vi "Move To Abs.vi"(8 "error in (no error)":errorcluster, 9 "Step In range":bool, 10 "Possition selector":T1(radio), 11 "Lifter_motor in":refnum<class "Lifter_motor.lvclass">) -> (0 "error out":errorcluster, 3 "Lifter_motor out":refnum<class "Lifter_motor.lvclass">)   [LabVIEW 2019, in "Lifter_motor.lvclass"]
uses:
  Lifter_motor.lvclass
  Lifter_motor.lvclass/Lifter_motor.ctl
  TCP Class/LifterTCP.lvclass
panel:
  out "Driver ACK?":bool
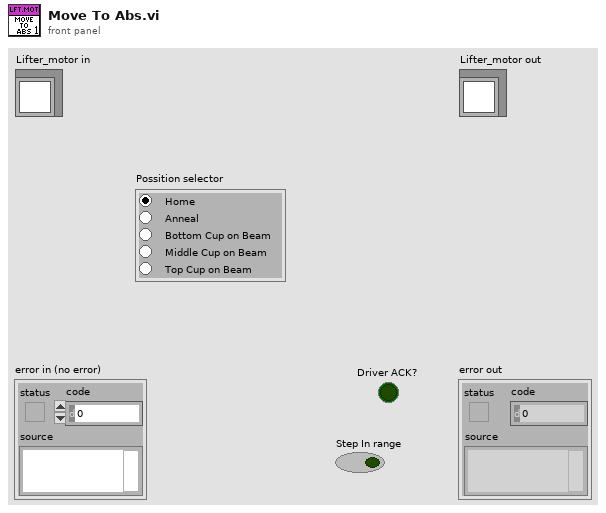
[diagram p1: front panel]
types:
  T1 = enum32{"Home", "Anneal", "Bottom Cup on Beam", "Middle Cup on Beam", "Top Cup on Beam"}
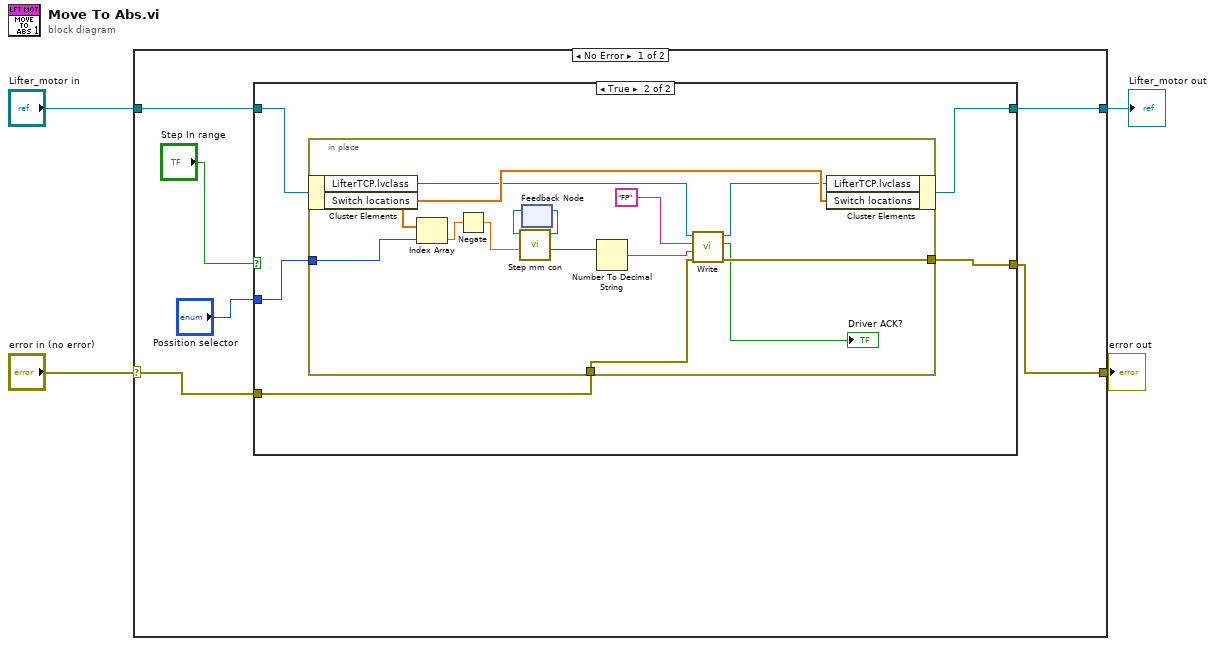
[diagram p0: block diagram]
diagram:
  n1 = case shown="No Error" "error in (no error)" {
    selector: "error in (no error)" -> [w7 w33]
    tunnel: [w6 w33] -> w3
    tunnel: "Lifter_motor in" -> [w9 w32]
    tunnel: [w8 w32] -> w1
    frame No Error {
      n2 = case shown="True" "Step In range" {
        tunnel: "Possition selector" -> [_ w17]
        tunnel: w9 -> [w12 w16]
        tunnel: [w12 w15] -> w8
        tunnel: w7 -> [w11 w14]
        tunnel: [w11 w13] -> w6
        frame False {
        }
        frame True {
          n3 = in-place {
            in-place-border: w17 -> [w30]
            in-place-border: w14 -> [w24]
            in-place-border: [w23] -> w13
            n4 = in-place-cluster #1(w16) -> ("LifterTCP.lvclass"=w28:refnum<class "LifterTCP.lvclass">, "Switch locations"=w31:dbl[])
            n5 = Index Array(array=w31, index=w30) -> (element=w29:dbl)
            n6 = Negate(x=w29) -> (-x=w19:dbl)
            n7 = feedback #2() -> (w20:refnum<class "Lifter_motor.lvclass">)  [unwired: 1 in]
            n8 = call "Step mm con.vi"("mm in"=w19, "Lifter_motor in"=w20) -> ("step out"=w18:i32, "Lifter_motor out"=w21:refnum<class "Lifter_motor.lvclass">)  [unwired: 6 in, 2 out]
            n9 = feedback-in #2(w21) -> ()
            n10 = Number To Decimal String(number=w18) -> (decimal integer string=w25:string)  [unwired: 1 in]
            n11 = call "Write.vi"("error in (no error)"=w24, "Parameter 2"=w25, "Parameter 1"="FP" ("string"), "LifterTCP in"=w28) -> ("error out"=w23:errorcluster, "Driver ACK?"=→"Driver ACK?":bool, "LifterTCP out"=w27:refnum<class "LifterTCP.lvclass">)  [unwired: 5 in]
            n12 = in-place-cluster #1("LifterTCP.lvclass"=w27, "Switch locations"=w31) -> (w15:refnum<class "Lifter_motor.lvclass">)
          }
        }
      }
    }
    frame Error {
    }
  }
  "error out" <- w3
  "Lifter_motor out" <- w1
